vi "DoubleSolenoidPulse_Example.vi"() -> ()   [LabVIEW 2019]
uses:
  <vilib>/Rock Robotics/WPI/Solenoid/WPI_SolenoidValue.ctl
  <vilib>/Rock Robotics/WPI/ThirdParty/JAS_Junk/TrajLib/VI/Util_GetTime_U32.vi
  <vilib>/Rock Robotics/WPI/ThirdParty/JAS_Junk/TrajLib/VI/Util_GetTime_U64.vi
  <vilib>/Rock Robotics/WPI/ThirdParty/JAS_Junk/TrajLib/Trajectory_Library.lvlib
panel:
  out "Solenoid Cmd":T1
  in  "Solenoid Pulse\nTime\nSeconds":dbl=1.0 format="%#_13g"
  in  "Robot Enabled":bool
  in  "Solenoid\\\nDemand":bool
  out "Waveform Chart":cluster{i16, i16, i16, i16}(graph)
  out "Solenoid\nReverse\nOutput":bool
  out "Solenoid\nForward\nOutput":bool
  # "DOUBLE SOLENOID PULSE HELPER"
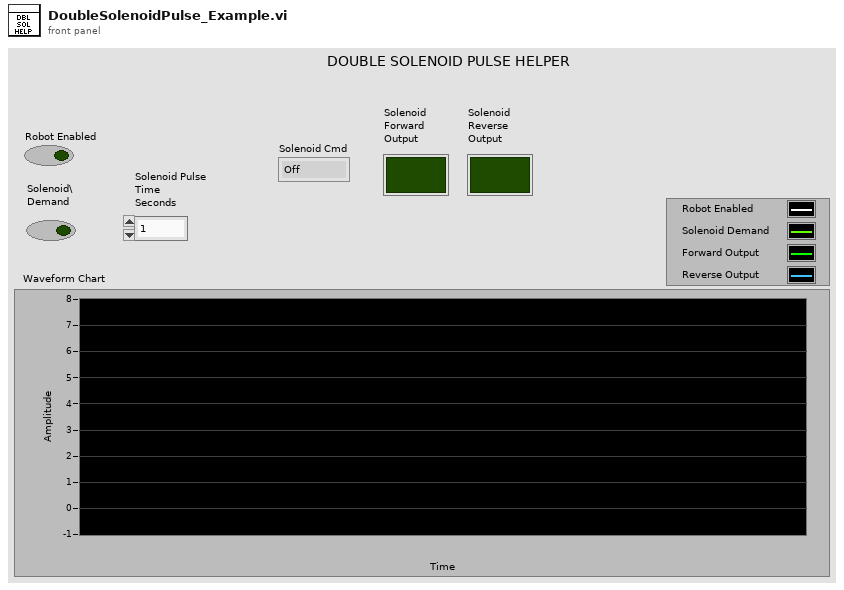
[diagram p1: front panel]
types:
  T1 = typedef "WPI_SolenoidValue.ctl" = enum16{"Off", "On", "Forward", "Reverse"}
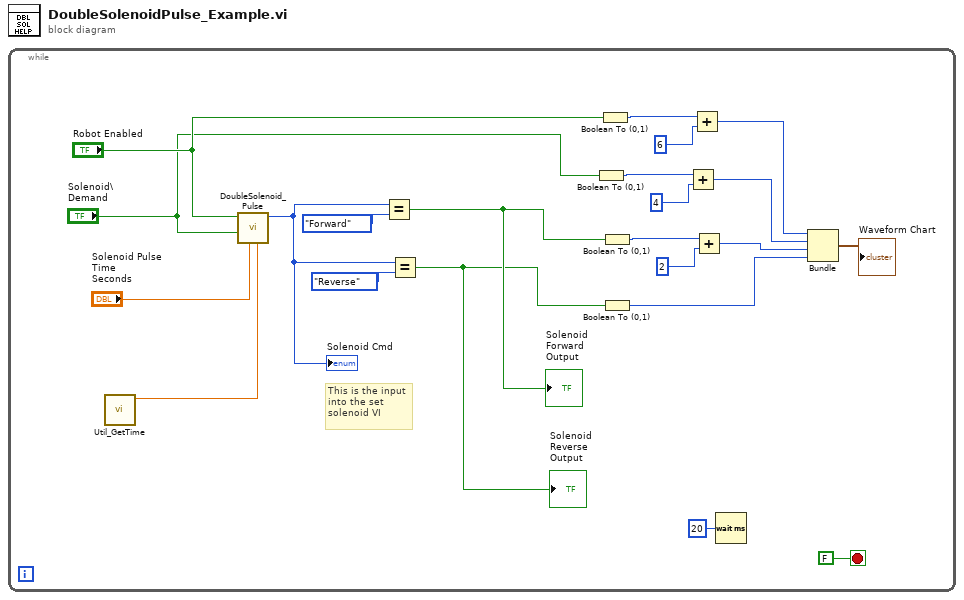
[diagram p0: block diagram]
diagram:
  n1 = while {
    stop <- FALSE stop-if-true
    # "This is the input\ninto the set \nsolenoid VI"
    n2 = call <vilib>:"Util_GetTime.vi"() -> ("FPGA_Time_Seconds"=w11:dbl)  [unwired: 9 in, 2 out]
    n3 = call <vilib>:"DoubleSolenoid_Pulse.vi"("Pass_Through_Time"=w11, "Solenoid Pulse\nTime\nSeconds"="Solenoid Pulse\nTime\nSeconds", "Solenoid Demand"="Solenoid\\\nDemand", "Robot Enabled"="Robot Enabled") -> ("Solenoid Cmd"=w12:T1)  [unwired: 7 in]
    "Solenoid Cmd" <- w12
    n4 = Equal?(x=w12, y=WPI_SolenoidValue."Forward") -> (x = y?=w3:bool)
    "Solenoid\nForward\nOutput" <- w3
    n5 = Equal?(x=w12, y=WPI_SolenoidValue."Reverse") -> (x = y?=w2:bool)
    "Solenoid\nReverse\nOutput" <- w2
    n6 = Boolean To (0,1)(Boolean="Solenoid\\\nDemand") -> (0, 1=w9:i16)
    n7 = Boolean To (0,1)(Boolean="Robot Enabled") -> (0, 1=w6:i16)
    n8 = Boolean To (0,1)(Boolean=w3) -> (0, 1=w18:i16)
    n9 = Boolean To (0,1)(Boolean=w2) -> (0, 1=w16:i16)
    n10 = Add(x=w9, y=i16 4) -> (x+y=w8:i16)
    n11 = Add(x=w6, y=i16 6) -> (x+y=w1:i16)
    n12 = Add(x=w18, y=i16 2) -> (x+y=w17:i16)
    n13 = Wait (ms)(milliseconds to wait=u32 20) -> ()  [unwired: 1 out]
    n14 = Bundle(w1, w8, w17, w16) -> (→"Waveform Chart":cluster{i16, i16, i16, i16})  [unwired: 1 in]
  }
